vi "get reservation property strings.vi"(10 "channel type":T1) -> (1 "notes":string, 2 "reservations":string, 3 "map":string)   [LabVIEW 2016]
uses:
  SubVIs/Channel Type.ctl
  FPGA Addon System Explorer.lvlib
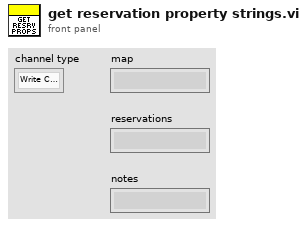
[diagram p1: front panel]
types:
  T1 = typedef "FPGA Addon System Explorer.lvlib/Channel Type.ctl" = enum16{"Write Channel", "Read Channel", "Write Waveform", "Read Waveform"}
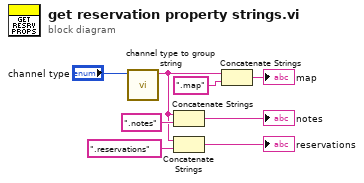
[diagram p0: block diagram]
diagram:
  n1 = call "channel type to group string.vi"("channel type"="channel type") -> ("FPGA.Controls"=w1:string)  [unwired: 10 in]
  n2 = Concatenate Strings(w1, ".notes" ("string")) -> (→"notes":string)
  n3 = Concatenate Strings(w1, ".reservations" ("string")) -> (→"reservations":string)
  n4 = Concatenate Strings(w1, ".map" ("string")) -> (→"map":string)
